vi "Find Aircraft COM Ports.vi"(8 "Error In":errorcluster) -> (0 "Error Out":errorcluster, 3 "Aircraft COM Port":refnum<visa-resource-name>)   [LabVIEW 2014]
panel:
  out "read buffer":string
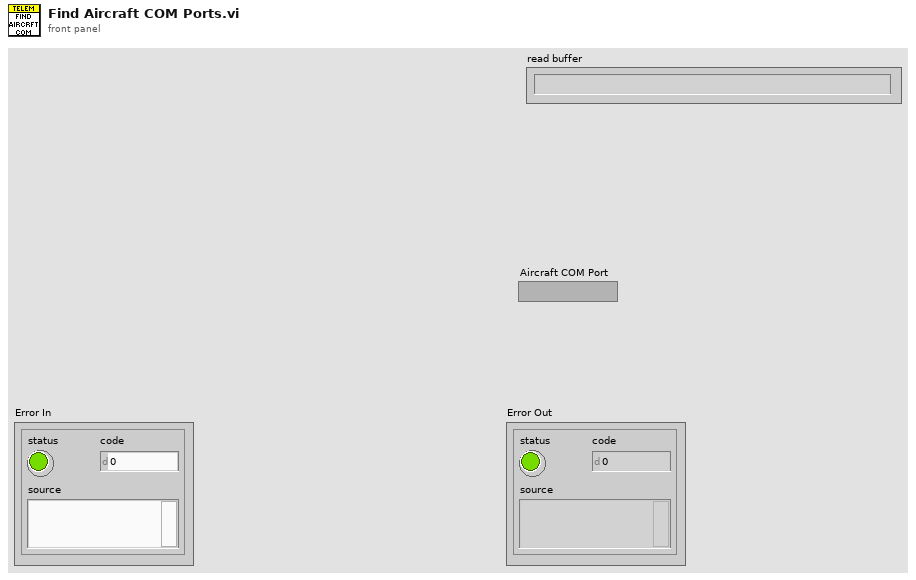
[diagram p1: front panel]
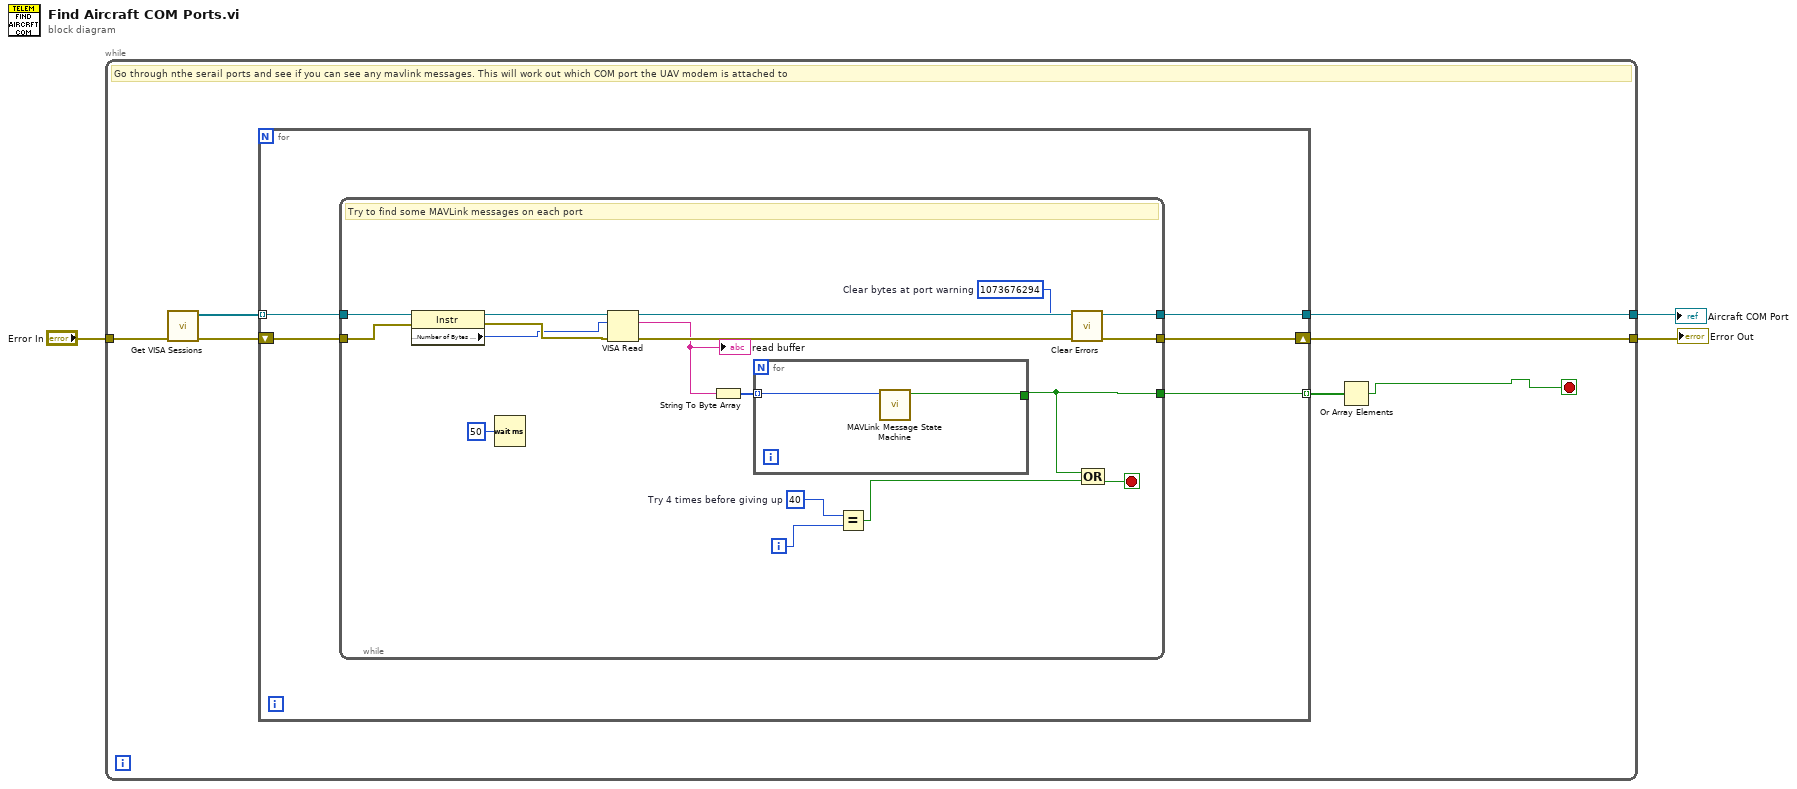
[diagram p0: block diagram]
diagram:
  n1 = while {
    tunnel: [w8] -> w1
    tunnel: "Error In" -> [w9]
    tunnel: [w7] -> w2
    stop <- w5 stop-if-true
    # "Go through nthe serail ports and see if you can see any mavlink messages. This will work out which COM port the UAV modem is attached to"
    n2 = call "Get VISA Sessions.vi"("Error In"=w9) -> ("Error Out"=w10:errorcluster, "Visa Sources"=w4:refnum<visa-resource-name>[])  [unwired: 9 in]
    n3 = for {
      tunnel: [w14] -> w8
      shift-right: [w13] -> w7
      shift-left: w10 -> [w15]
      tunnel: w4 -> [w12] mode=indexing
      tunnel: [w11] -> w6 mode=indexing
      n4 = while {
        tunnel: w12 -> [w31]
        tunnel: w15 -> [w30]
        tunnel: [w22] -> w14
        tunnel: [w21] -> w11
        tunnel: [w18] -> w13
        i -> [w26]
        stop <- w23 stop-if-true
        w17 = 1073676294  # Clear bytes at port warning
        w25 = 40  # Try 4 times before giving up
        # "Try to find some MAVLink messages on each port"
        n5 = property class="Instr"(reference=w31, error in=w30) -> (reference out=w29:refnum<visa-resource-name>, error out=w28:errorcluster, "Serial Settings:Number of Bytes at Serial Port"=w20:u32)
        n6 = Wait (ms)(milliseconds to wait=u32 50) -> ()  [unwired: 1 out]
        n7 = VISA Read(VISA resource name=w29, byte count=w20, error in (no error)=w28) -> (VISA resource name out=w22:refnum<visa-resource-name>, read buffer=w16:string, error out=w19:errorcluster)  [unwired: 1 out]
        "read buffer" <- w16
        n8 = String To Byte Array(string=w16) -> (unsigned byte array=w32:u8[])
        n9 = for {
          tunnel: w32 -> [w34] mode=indexing
          tunnel: [w33] -> w21
          n10 = call "MAVLink Message State Machine.vi"("Incoming Bytes"=w34) -> ("Message Complete"=w33:bool)  [unwired: 7 in, 3 out]
        }
        n11 = Equal?(x=w25, y=w26) -> (x = y?=w24:bool)
        n12 = call <vilib>:"Clear Errors.vi"("error in (no error)"=w19, "specific error code to clear (0: all)"=w17) -> ("error out"=w18:errorcluster)  [unwired: 4 in, 1 out]
        n13 = Compound Arithmetic op=OR(w21, w24) -> (w23:bool)
      }
    }
    n14 = Or Array Elements(Boolean array=w6) -> (logical OR=w5:bool)
  }
  "Aircraft COM Port" <- w1
  "Error Out" <- w2
